vi "Auto_Path Tracking_KBS.vi"() -> ()   [LabVIEW 2020]
uses:
  <vilib>/Utility/file.llb/Read Delimited Spreadsheet (DBL).vi
  <vilib>/Instr/_visa.llb/VISA Configure Serial Port (Instr).vi
panel:
  out "Tracking_Error(m)":dbl
  out "TM_X(lat)":dbl format="%-#_10g M"
  out "TM_Y(long)":dbl format="%-#_10g M"
  out "F9P_Data_GPGGA_Raw":string
  out "GPS_KHP":dbl
  out "Heading_T":dbl
  out "Heading_M":dbl
  out "F9P GPS Data":T1
  in  "COM":refnum<visa-resource-name>="COM4"
  in  "?":enum32{"State", "ETC"}(tab)
  in  "stop":bool
  in  "file path (dialog if empty)":path caption="RDDF"
  out "XY Graph":T2(graph)
  in  "Refresh":bool
  in  "A/M":bool=TRUE
  in  "Serial Name":refnum<visa-resource-name>="COM8"
  out "ERP_Serial_DATA(RAW)":string
  in  "Vel":dbl=4.0 format="%#_13g"
  out "Index(near vehicle)":i32
  out "WP_no.":i32
  out "x_lat_path":dbl[](array[numeric])
  out "y_long_path":dbl[](array[numeric])
  out "vel. path":dbl[](array[numeric])
  out "Path_Vel_arr":dbl[](array[numeric])
  out "Path_long_arr":dbl[](array[numeric])
  out "Path_lat_arr":dbl[](array[numeric])
  out "ERP_Receive":T3
  out "Steer_CMD(Deg)":dbl
  out "CMD_2_ERP":T4
  out "Brake":u8
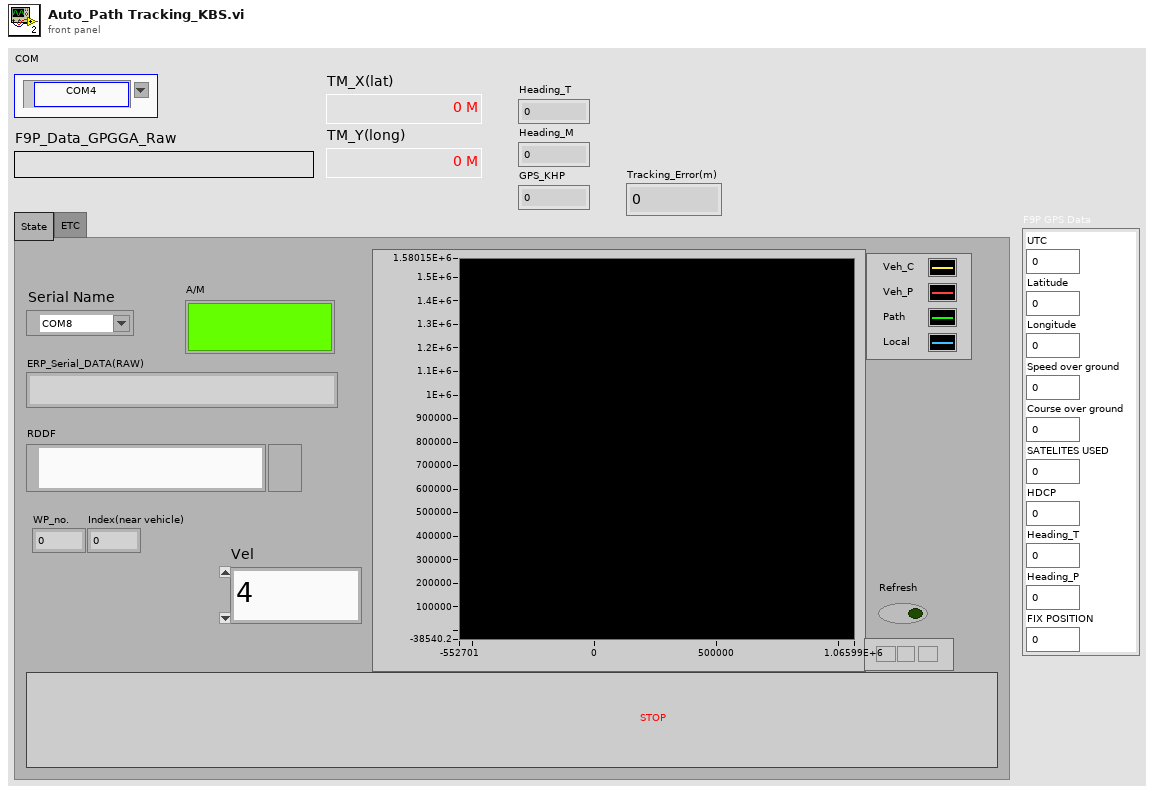
[diagram p1: front panel]
types:
  T1 = cluster{"UTC":dbl, "Latitude":dbl, "Longitude":dbl, "Speed over ground":dbl, "Course over ground":dbl, "SATELITES USED":i32, "HDCP":dbl, "Heading_T":dbl, "Heading_P":dbl, "FIX POSITION":i32}
  T2 = cluster{"y_long_path":dbl[], "x_lat_path":dbl[]}[]
  T3 = cluster{"AorM":u8, "E-Stop":u8, "F_B":u8, "Speed":u16, "Steer":i16, "Brake":u8, "Encoder":u8, "Encoder 2":u8, "Encoder 3":u8, "Encoder 4":u8, "ALIVE":u8, "ETX_0":u8, "ETX_0 2":u8}
  T4 = cluster{"F/B":u8, "Speed":u16, "Steer":i16, "A/M":u8, "Brake":u8}
  T5 = cluster{"Path_long_arr":dbl[], "Path_lat_arr":dbl[]}
  T6 = cluster{"Path_long_arr":dbl[], "Path_lat_arr":dbl[]}[]
  T7 = cluster{"S":u8, "T":u8, "X":u8, "AorM":u8, "E-Stop":u8, "F_B":u8, "Speed":u16, "Steer":i16, "Brake":u8, "ALIVE":u8, "ETX_0":u8, "ETX_0 2":u8}
  T8 = cluster{"UTC":dbl, "Latitude":dbl, "N/S":i8, "Longitude":dbl, "N/S":i8, "FIX POSITION":i32, "SATELITES USED":i32, "HDCP":dbl}
  T9 = cluster{"UTC":dbl, "N/S":i8, "Latitude":dbl, "N/S 2":i8, "Longitude":dbl, "N/S 3":i8, "Speed over ground":dbl, "Course over ground":dbl}
  T10 = cluster{"Heading_T":dbl, "T":i8, "Heading_M":dbl, "M":i8, "G_Speed_Knote":dbl, "N":i8, "G_Speed_KPH":dbl}
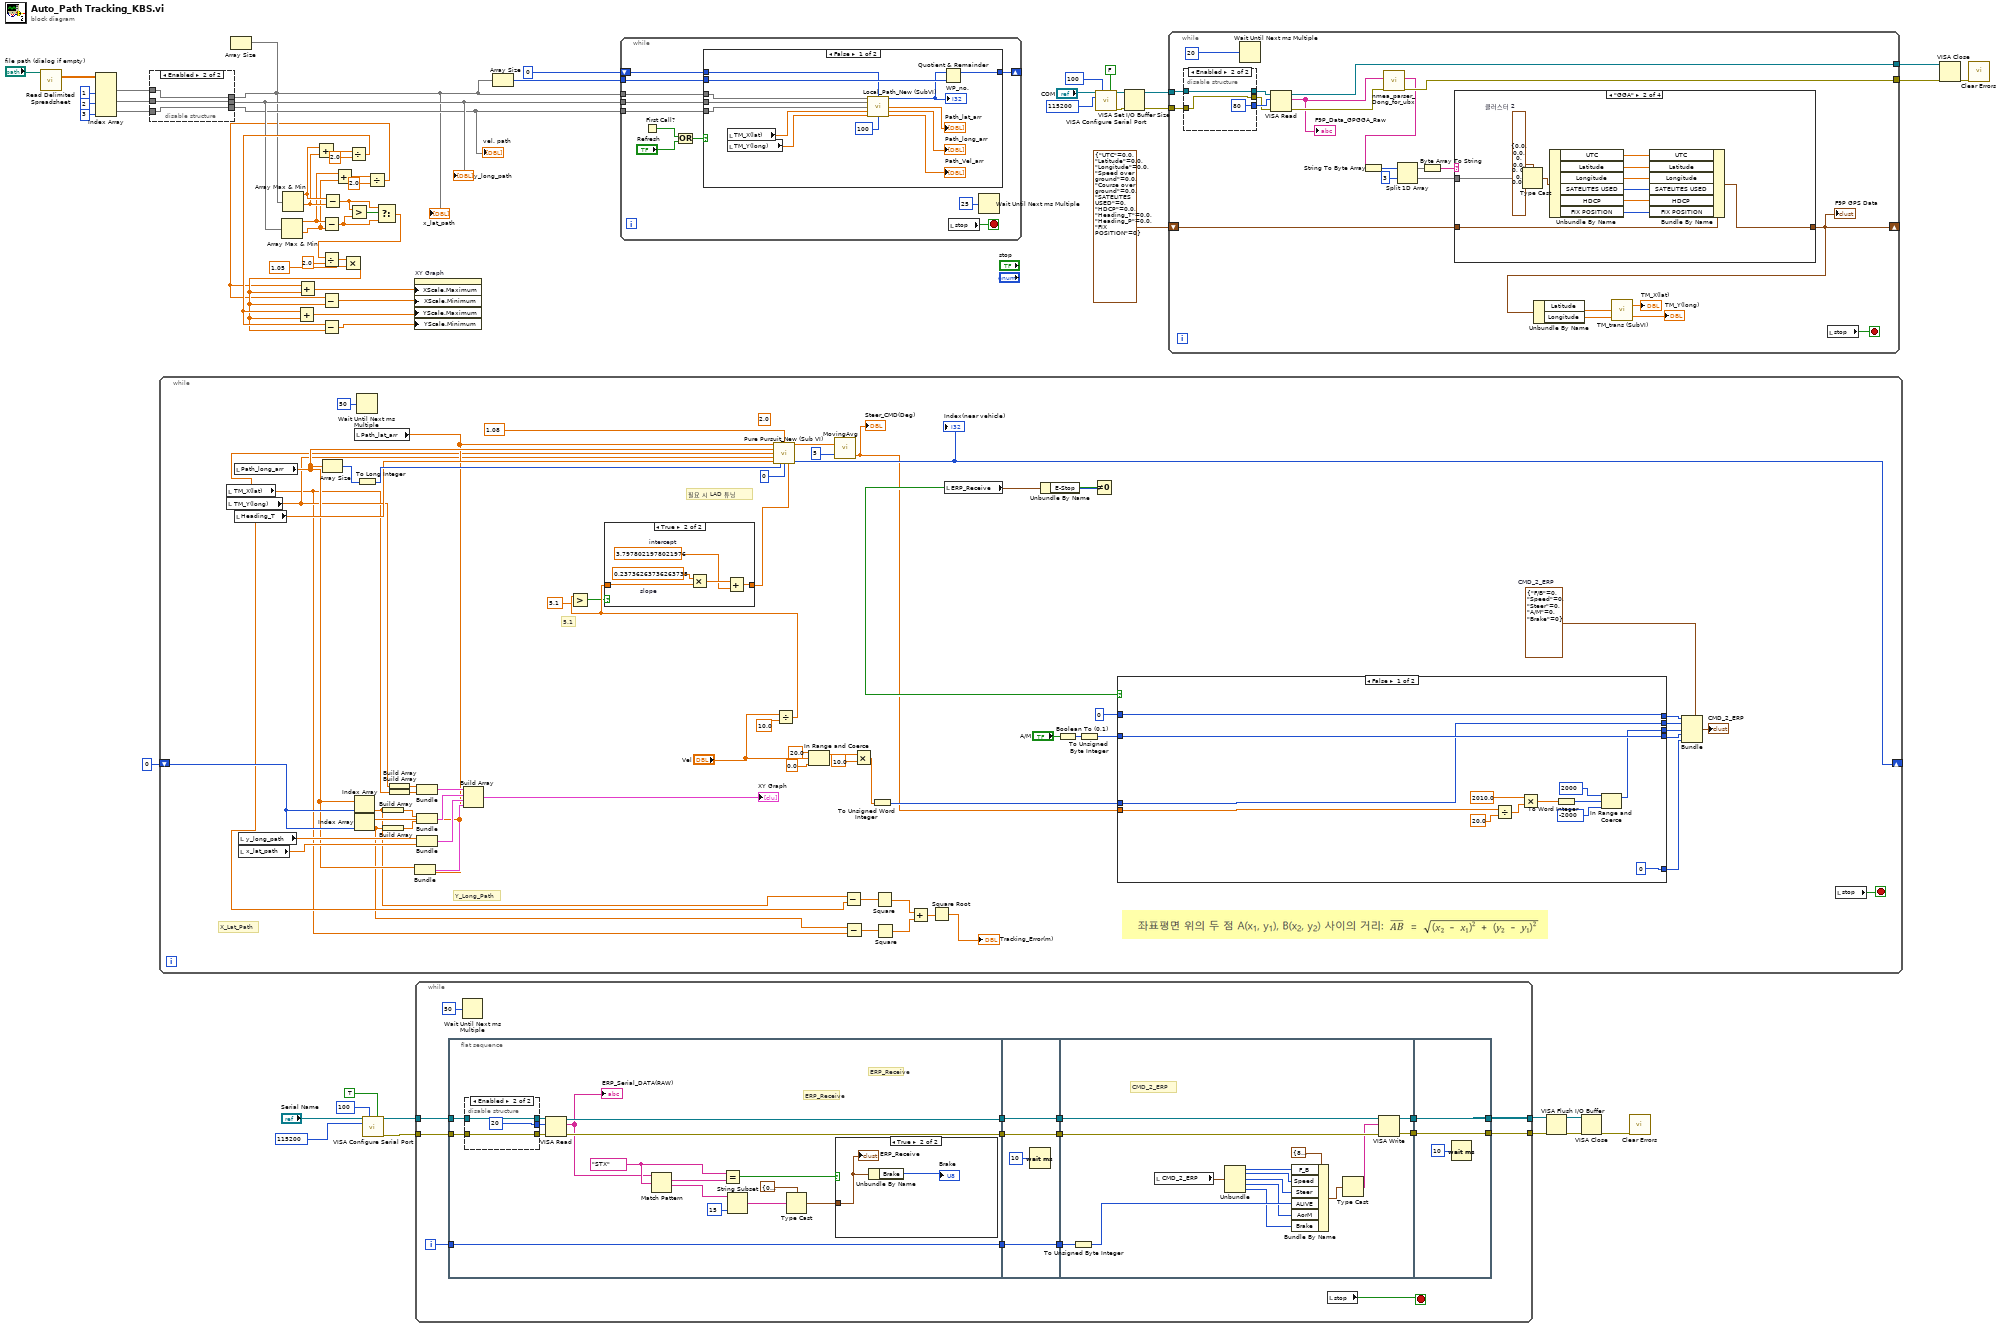
[diagram p0: block diagram]
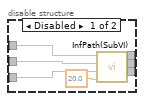
[diagram p2: hidden frame]
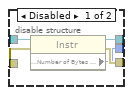
[diagram p3: hidden frame]
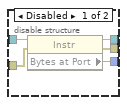
[diagram p5: hidden frame]
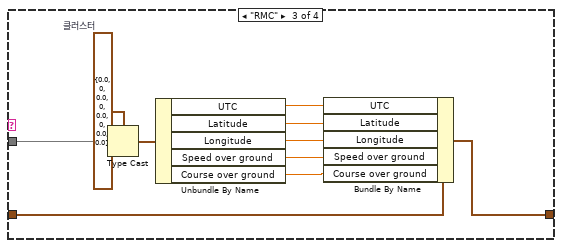
[diagram p7: hidden frame]
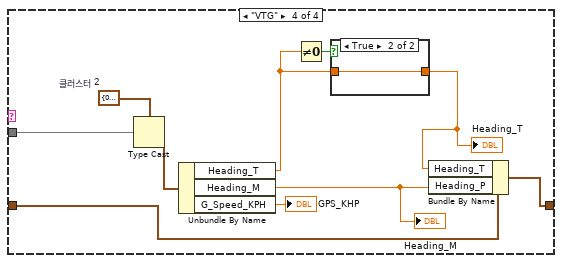
[diagram p8: hidden frame]
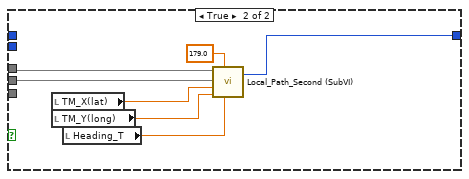
[diagram p10: hidden frame]
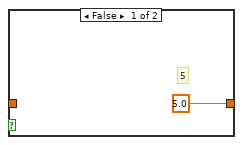
[diagram p11: hidden frame]
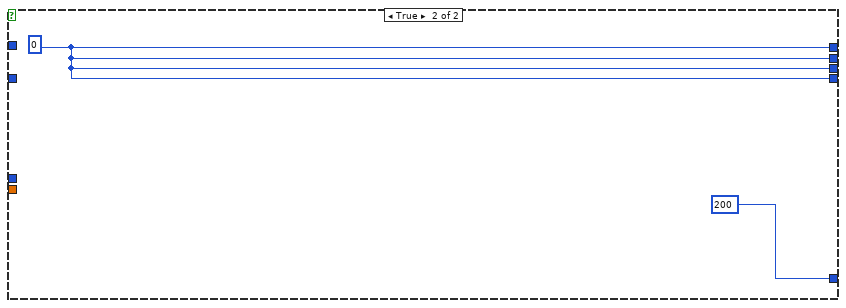
[diagram p12: hidden frame]
diagram:
  n1 = call-poly <vilib>:"Read Delimited Spreadsheet.vi"("file path (dialog if empty)"="file path (dialog if empty)") -> ("all rows"=w27:dbl[][])  [unwired: 9 in, 5 out]
  n2 = Index Array(array=w27, index (col) #1=1 ("비활성화된 인덱스 (열)"), index (col) #2=2 ("인덱스 (열)"), index (col) #3=3 ("인덱스 (열)")) -> (element #1=w56:dbl[], element #2=w55:dbl[], element #3=w54:dbl[])  [unwired: 3 in]
  n3 = disable-structure shown="Enabled" {
    disable-tunnel: w56 -> [w66 w69]
    disable-tunnel: w55 -> [w65 w68]
    disable-tunnel: w54 -> [w64 w67]
    disable-tunnel: [w63 w68] -> w31
    disable-tunnel: [w62 w67] -> w29
    disable-tunnel: [w61 w69] -> w28
    frame Disabled {
      n4 = call "InfPath(SubVI).vi"("Mod dist."=20.0, "vel."=w64, "y_long"=w65, "x_lat"=w66) -> ("vel. path"=w62:dbl[], "y_long_path"=w63:dbl[], "x_lat_path"=w61:dbl[])  [unwired: 1 out]
    }
    frame Enabled {
    }
  }
  "x_lat_path" <- w28
  "y_long_path" <- w31
  "vel. path" <- w29
  n5 = while {
    shift-right: [w117] -> _
    shift-left: 0 -> [w114]
    stop <- w123 stop-if-true
    w89 = T4 {"F/B"=0, "Speed"=0, "Steer"=0, "A/M"=0, "Brake"=0}  # CMD_2_ERP
    (unwired) 2.0 ("L")
    # "5.1"
    # "X_Lat_Path"
    # "Y_Long_Path"
    # "필요 시 LAD 튜닝"
    n6 = local read "TM_X(lat)"() -> (w83:dbl)
    n7 = local read "TM_Y(long)"() -> (w84:dbl)
    n8 = local read "Path_long_arr"() -> (w86:dbl[])
    n9 = local read "Heading_T"() -> (w110:dbl)
    n10 = local read "y_long_path"() -> (w94:dbl[])
    n11 = local read "x_lat_path"() -> (w93:dbl[])
    n12 = Array Size(array=w86) -> (size(s)=w118:i32)
    n13 = local read "Path_lat_arr"() -> (w85:dbl[])
    n14 = Index Array(array=w86, index=w114) -> (element=w74:dbl)
    n15 = Index Array(array=w85, index=w114) -> (element=w73:dbl)
    n16 = Wait Until Next ms Multiple(millisecond multiple=u32 50 ("ms 배수")) -> ()  [unwired: 1 out]
    n17 = To Long Integer(number=w118) -> (32bit integer=w116:i32)
    n18 = Build Array(w74) -> (w125:dbl[])
    n19 = Build Array(w73) -> (w124:dbl[])
    n20 = Build Array(w84) -> (w127:dbl[])
    n21 = Build Array(w83) -> (w126:dbl[])
    n22 = Bundle("Path_long_arr"=w86, "Path_lat_arr"=w85) -> (w106:T5)  [unwired: 1 in]
    n23 = Bundle(w127, w126) -> (w112:cluster{dbl[], dbl[]})  [unwired: 1 in]
    n24 = Bundle(w125, w124) -> (w111:cluster{dbl[], dbl[]})  [unwired: 1 in]
    n25 = Bundle("y_long_path"=w94, "x_lat_path"=w93) -> (w113:cluster{"y_long_path":dbl[], "x_lat_path":dbl[]})  [unwired: 1 in]
    n26 = Build Array(w112, w111, w113, w106) -> (→"XY Graph":T6)
    n27 = Divide(x="Vel", y=10.0) -> (x/y=w107:dbl)
    n28 = Greater?(x=w107, y=5.1) -> (0:w72:bool)
    n29 = case shown="True" w72 {
      tunnel: w107 -> [_ w133]
      tunnel: [5.0 w132] -> w109
      frame False {
        # "5"
      }
      frame True {
        w134 = 3.7978021978021976  # intercept
        w136 = 0.23736263736263735  # slope
        n30 = Multiply(x=w136, y=w133) -> (x*y=w135:dbl)
        n31 = Add(x=w135, y=w134) -> (x+y=w132:dbl)
      }
    }
    n32 = call "Pure Pursuit_New (Sub VI).vi"("x_lat_path"=w85, "L"=1.08, "y_long_path"=w86, "X_Current"=w83, "Y_Current"=w84, "Heading_Current"=w110, "#pnt"=w116, "WP no_pre"=0, "LAD"=w109) -> ("Steer_CMD(Deg)"=w82:dbl, "Index(near vehicle)"=w117:i32)  [unwired: 5 in]
    "Index(near vehicle)" <- w117
    n33 = In Range and Coerce(upper limit=20.0 ("상위 리미트"), x="Vel", lower limit=0.0 ("하위 리미트")) -> (coerced(x)=w98:dbl)  [unwired: 1 out]
    n34 = call "MovingAvg.vi"("입력"=w82, "이동평균을 구할 자료의 개수"=u16 5) -> ("이동평균"=w70:dbl)  [unwired: 2 out]
    "Steer_CMD(Deg)" <- w70
    n35 = Subtract(x=w74, y=w84) -> (x-y=w79:dbl)
    n36 = Subtract(x=w73, y=w83) -> (x-y=w78:dbl)
    n37 = Multiply(x=w98, y=10.0) -> (x*y=w96:dbl)
    n38 = To Unsigned Word Integer(number=w96) -> (unsigned 16bit integer=w102:u16)
    n39 = Square(x=w79) -> (x^2=w77:dbl)
    n40 = Square(x=w78) -> (x^2=w76:dbl)
    n41 = Add(x=w77, y=w76) -> (x+y=w75:dbl)
    n42 = Square Root(x=w75) -> (sqrt(x)=→"Tracking_Error(m)":dbl)
    n43 = local read "ERP_Receive"() -> (w120:T3)
    n44 = Unbundle By Name(w120) -> ("E-Stop"=w121:u8)
    n45 = Boolean To (0,1)(Boolean="A/M") -> (0, 1=w105:i16)
    n46 = To Unsigned Byte Integer(number=w105) -> (unsigned 8bit integer=w87:u8)
    n47 = Not Equal To 0?(x=w121) -> (x != 0?=w101:bool)
    n48 = case shown="False" w101 {
      tunnel: u8 0 -> [w149 _]
      tunnel: [w149 w151] -> w130
      tunnel: [w146 w151] -> w129
      tunnel: [w138 w151] -> w128
      tunnel: [w148 w151] -> w104
      tunnel: w87 -> [w148 _]
      tunnel: w70 -> [w147 _]
      tunnel: w102 -> [w146 _]
      tunnel: [u8 0 u8 200] -> w90
      frame False {
        n49 = Divide(x=w147, y=20.0) -> (x/y=w144:dbl)
        n50 = Multiply(x=2010.0, y=w144) -> (x*y=w143:dbl)
        n51 = To Word Integer(number=w143) -> (16bit integer=w145:i16)
        n52 = In Range and Coerce(upper limit=i16 2000 ("상위 리미트"), x=w145, lower limit=i16 -2000 ("하위 리미트")) -> (coerced(x)=w138:i16)  [unwired: 1 out]
      }
      frame True {
        w151 = u8 0
      }
    }
    n53 = Bundle(cluster=w89, "F/B"=w130, "Speed"=w129, "Steer"=w128, "A/M"=w104, "Brake"=w90) -> (→"CMD_2_ERP":T4)
    n54 = local read "stop"() -> (w123:bool)
  }
  n55 = Array Size(array=w28) -> ()  [unwired: 1 out]
  n56 = Array Max & Min(array=w31) -> (max value=w42:dbl, min value=w41:dbl)  [unwired: 2 out]
  n57 = Array Max & Min(array=w28) -> (max value=w48:dbl, min value=w47:dbl)  [unwired: 2 out]
  n58 = Add(x=w48, y=w47) -> (x+y=w45:dbl)
  n59 = Subtract(x=w42, y=w41) -> (x-y=w51:dbl)
  n60 = Subtract(x=w48, y=w47) -> (x-y=w52:dbl)
  n61 = Add(x=w42, y=w41) -> (x+y=w44:dbl)
  n62 = Divide(x=w45, y=2.0) -> (x/y=w38:dbl)
  n63 = Greater?(x=w52, y=w51) -> (0:w53:bool)
  n64 = call-poly "VISA Configure Serial Port"("VISA resource name"="Serial Name", "timeout (10sec)"=u32 100, "Enable Termination\nChar (T)"=TRUE ("Enable Termination\nChar (T)"), "baud rate (9600)"=u32 115200) -> ("VISA resource name out"=w3:refnum<visa-resource-name>, "error out"=w2:errorcluster)  [unwired: 10 in]
  n65 = Divide(x=w44, y=2.0) -> (x/y=w25:dbl)
  n66 = Select(t=w52, s=w53, f=w51) -> (s? t:f=w49:dbl)
  n67 = Divide(x=w49, y=2.0) -> (x/y=w40:dbl)
  n68 = Multiply(x=w40, y=1.05) -> (x*y=w37:dbl)
  n69 = Add(x=w38, y=w37) -> (x+y=w35:dbl)
  n70 = Add(x=w25, y=w37) -> (x+y=w33:dbl)
  n71 = Subtract(x=w25, y=w37) -> (x-y=w34:dbl)
  n72 = Subtract(x=w38, y=w37) -> (x-y=w36:dbl)
  n73 = property on="XY Graph" class="XYGraph (strict)"("XScale.Maximum"=w33, "XScale.Minimum"=w34, "YScale.Maximum"=w35, "YScale.Minimum"=w36) -> ()  [unwired: 2 in, 2 out]
  n74 = while {
    tunnel: w3 -> [w165]
    tunnel: w2 -> [w164]
    tunnel: [w162] -> w5
    tunnel: [w161] -> w4
    i -> [w163]
    stop <- w154 stop-if-true
    n75 = flat-sequence {
      tunnel: w165 -> [w183]
      tunnel: w164 -> [w182]
      tunnel: [w181] -> w160
      tunnel: [w180] -> w158
      tunnel: w163 -> [w179]
      tunnel: [w179] -> w156
      tunnel: w160 -> [w197]
      tunnel: [w197] -> w159
      tunnel: w158 -> [w196]
      tunnel: [w196] -> w157
      tunnel: w156 -> [w195]
      tunnel: [w195] -> w155
      tunnel: w159 -> [w210]
      tunnel: w157 -> [w209]
      tunnel: w155 -> [w207]
      tunnel: [w206] -> w153
      tunnel: [w205] -> w152
      tunnel: [w214] -> w161
      tunnel: [w215] -> w162
      tunnel: w153 -> [w215]
      tunnel: w152 -> [w214]
      frame #0 {
        w173 = "STX" ("검색 문자열/문자 (-)")
        # "ERP_Receive"
        # "ERP_Receive"
        n76 = disable-structure shown="Enabled" {
          disable-tunnel: w183 -> [w188 w190]
          disable-tunnel: w182 -> [w187 w191]
          disable-tunnel: [w186 w191] -> w178
          disable-tunnel: [w185 u32 20 ("timeout (10sec)")] -> w177
          disable-tunnel: [w184 w190] -> w176
          frame Disabled {
            n77 = property class="Instr"(reference=w188, error in=w187) -> (reference out=w184:refnum<visa-resource-name>, error out=w186:errorcluster, "Serial Settings:Number of Bytes at Serial Port"=w185:u32)
          }
          frame Enabled {
          }
        }
        n78 = VISA Read(VISA resource name=w176, byte count=w177, error in (no error)=w178) -> (VISA resource name out=w181:refnum<visa-resource-name>, read buffer=w171:string, error out=w180:errorcluster)  [unwired: 1 out]
        "ERP_Serial_DATA(RAW)" <- w171
        n79 = Match Pattern(string=w171, regular expression=w173) -> (match substring=w172:string, after substring=w175:string)  [unwired: 1 in, 2 out]
        n80 = Equal?(x=w173, y=w172) -> (x = y?=w170:bool)
        n81 = String Subset(string=w175, length (rest)=15 ("길이(나머지)")) -> (substring=w169:string)  [unwired: 1 in]
        n82 = Type Cast(type=T3 {"AorM"=0, "E-Stop"=0, "F_B"=0, "Speed"=0, "Steer"=0, "Brake"=0, "Encoder"=0, "Encoder 2"=0, "Encoder 3"=0, "Encoder 4"=0, "ALIVE"=0, "ETX_0"=13, "ETX_0 2"=10}, x=w169) -> (*(type *) &x=w168:T3)
        n83 = case shown="True" w170 {
          tunnel: w168 -> [_ w193]
          frame False {
          }
          frame True {
            n84 = Unbundle By Name(w193) -> ("Brake"=→"Brake":u8)
            "ERP_Receive" <- w193
          }
        }
      }
      frame #1 {
        n85 = Wait (ms)(milliseconds to wait=u32 10 ("대기 시간(ms)")) -> ()  [unwired: 1 out]
      }
      frame #2 {
        # "CMD_2_ERP"
        n86 = To Unsigned Byte Integer(number=w207) -> (unsigned 8bit integer=w212:u8)
        n87 = local read "CMD_2_ERP"() -> (w199:T4)
        n88 = Unbundle(w199) -> ("F/B"=w204:u8, "Speed"=w203:u16, "Steer"=w202:i16, "A/M"=w200:u8, "Brake"=w198:u8)
        n89 = Bundle By Name(cluster=T7 {"S"=83, "T"=84, "X"=88, "AorM"=0, "E-Stop"=0, "F_B"=0, "Speed"=0, "Steer"=0, "Brake"=0, "ALIVE"=0, "ETX_0"=13, "ETX_0 2"=10}, "F_B"=w204, "Speed"=w203, "Steer"=w202, "ALIVE"=w212, "AorM"=w200, "Brake"=w198) -> (w211:T7)
        n90 = Type Cast(x=w211) -> (*(type *) &x=w208:string)  [unwired: 1 in]
        n91 = VISA Write(VISA resource name=w210, write buffer=w208, error in (no error)=w209) -> (VISA resource name out=w206:refnum<visa-resource-name>, error out=w205:errorcluster)  [unwired: 1 out]
      }
      frame #3 {
        n92 = Wait (ms)(milliseconds to wait=u32 10 ("대기 시간(ms)")) -> ()  [unwired: 1 out]
      }
    }
    n93 = Wait Until Next ms Multiple(millisecond multiple=u32 50 ("ms 배수")) -> ()  [unwired: 1 out]
    n94 = local read "stop"() -> (w154:bool)
  }
  n95 = Array Size(array=w28) -> (size(s)=w30:i32)
  n96 = while {
    tunnel: w28 -> [w225]
    tunnel: w31 -> [w224]
    tunnel: w29 -> [w222]
    tunnel: w30 -> [w221]
    shift-right: [w220] -> _
    shift-left: 0 ("Index0") -> [w223]
    stop <- w226 stop-if-true
    n97 = First Call?() -> (First Call?: T/F=w218:bool)
    n98 = Or(x=w218, y="Refresh") -> (x .or. y?=w219:bool)
    n99 = case shown="False" w219 {
      tunnel: w225 -> [w227 w246]
      tunnel: w224 -> [w229 w245]
      tunnel: w223 -> [w234 _]
      tunnel: w222 -> [w228 _]
      tunnel: w221 -> [w238 _]
      tunnel: [w239 w240] -> w220
      frame False {
        n100 = local read "TM_X(lat)"() -> (w237:dbl)
        n101 = local read "TM_Y(long)"() -> (w236:dbl)
        n102 = call "Local_Path_New (SubVI).vi"("x_lat_arr"=w227, "WP no_pre"=w234, "y_long_arr"=w229, "vel_arr"=w228, "x_lat_c"=w237, "y_long_c"=w236, "# of pnt"=100) -> ("INDEX(Near Point)"=w230:i32, "Lat(Local)"=→"Path_lat_arr":dbl[], "Long(Local)"=→"Path_long_arr":dbl[], "Vel(Local)"=→"Path_Vel_arr":dbl[])  [unwired: 5 in]
        "WP_no." <- w230
        n103 = Quotient & Remainder(x=w230, y=w238) -> (x-y*floor(x/y)=w239:i32)  [unwired: 1 out]
      }
      frame True {
        n104 = local read "TM_X(lat)"() -> (w244:dbl)
        n105 = local read "TM_Y(long)"() -> (w243:dbl)
        n106 = local read "Heading_T"() -> (w242:dbl)
        n107 = call "Local_Path_Second (SubVI).vi"("heading_deg"=w242, "heading_limit"=179.0, "y_long"=w243, "x_lat"=w244, "Y_long_path"=w245, "X_lat_path"=w246) -> ("Index(near vehicle)"=w240:i32)  [unwired: 1 out]
      }
    }
    n108 = local read "stop"() -> (w226:bool)
    n109 = Wait Until Next ms Multiple(millisecond multiple=u32 25) -> ()  [unwired: 1 out]
  }
  n110 = call-poly "VISA Configure Serial Port"("VISA resource name"="COM", "timeout (10sec)"=u32 100, "Enable Termination\nChar (T)"=FALSE ("Enable Termination\nChar (T)"), "baud rate (9600)"=u32 115200 ("baud rate")) -> ("VISA resource name out"=w20:refnum<visa-resource-name>, "error out"=w19:errorcluster)  [unwired: 10 in]
  n111 = VISA Set I/O Buffer Size(VISA resource name=w20, error in (no error)=w19) -> (VISA resource name out=w15:refnum<visa-resource-name>, error out=w14:errorcluster)  [unwired: 2 in]
  n112 = while {
    shift-right: [w261] -> _
    shift-left: T1 {"UTC"=0.0, "Latitude"=0.0, "Longitude"=0.0, "Speed over ground"=0.0, "Course over ground"=0.0, "SATELITES USED"=0, "HDCP"=0.0, "Heading_T"=0.0, "Heading_P"=0.0, "FIX POSITION"=0} ("Garmin GPS Data") -> [w269]
    tunnel: w15 -> [w253]
    tunnel: w14 -> [w251]
    tunnel: [w262] -> w18
    tunnel: [w268] -> w17
    stop <- w248 stop-if-true
    n113 = disable-structure shown="Enabled" {
      disable-tunnel: [w274 u32 80 ("Bytes at Port")] -> w254
      disable-tunnel: w253 -> [w273 w276]
      disable-tunnel: [w272 w276] -> w252
      disable-tunnel: w251 -> [w271 w275]
      disable-tunnel: [w270 w275] -> w250
      frame Disabled {
        n114 = property class="Instr"(reference=w273, error in=w271) -> (reference out=w272:refnum<visa-resource-name>, error out=w270:errorcluster, "Bytes at Port"=w274:u32)
      }
      frame Enabled {
      }
    }
    n115 = Wait Until Next ms Multiple(millisecond multiple=u32 20 ("타임아웃(ms) (-1)")) -> ()  [unwired: 1 out]
    n116 = VISA Read(VISA resource name=w252, byte count=w254, error in (no error)=w250) -> (VISA resource name out=w262:refnum<visa-resource-name>, read buffer=w263:string, error out=w267:errorcluster)  [unwired: 1 out]
    "F9P_Data_GPGGA_Raw" <- w263
    n117 = call "nmea_parser_Dong_for_ubx.vi"("error in"=w267, "INPUT"=w263) -> ("error out"=w268:errorcluster, "output"=w255:string)  [unwired: 8 in]
    n118 = String To Byte Array(string=w255) -> (unsigned byte array=w259:u8[])
    n119 = Split 1D Array(array=w259, index=3) -> (first subarray=w258:u8[], second subarray=w257:u8[])
    n120 = Byte Array To String(unsigned byte array=w258) -> (string=w256:string)
    n121 = case shown="\"GGA\"" w256 {
      tunnel: w257 -> [_ w289 w297 w309]
      tunnel: w269 -> [w278 w285 w296 w305]
      tunnel: [w278 w284 w295 w306] -> w261
      frame Default {
      }
      frame "GGA" {
        w287 = T8 {"UTC"=0.0, "Latitude"=0.0, "N/S"=0, "Longitude"=0.0, "N/S"=0, "FIX POSITION"=0, "SATELITES USED"=0, "HDCP"=0.0}  # 클러스터 2
        n122 = Type Cast(type=w287, x=w289) -> (*(type *) &x=w288:T8)
        n123 = Unbundle By Name(w288) -> ("UTC"=w286:dbl, "Latitude"=w283:dbl, "Longitude"=w282:dbl, "SATELITES USED"=w281:i32, "HDCP"=w280:dbl, "FIX POSITION"=w279:i32)
        n124 = Bundle By Name(cluster=w285, "UTC"=w286, "Latitude"=w283, "Longitude"=w282, "SATELITES USED"=w281, "HDCP"=w280, "FIX POSITION"=w279) -> (w284:T1)
      }
      frame "RMC" {
        w299 = T9 {"UTC"=0.0, "N/S"=0, "Latitude"=0.0, "N/S 2"=0, "Longitude"=0.0, "N/S 3"=0, "Speed over ground"=0.0, "Course over ground"=0.0}  # 클러스터
        n125 = Type Cast(type=w299, x=w297) -> (*(type *) &x=w298:T9)
        n126 = Unbundle By Name(w298) -> ("UTC"=w294:dbl, "Latitude"=w293:dbl, "Longitude"=w292:dbl, "Speed over ground"=w291:dbl, "Course over ground"=w290:dbl)
        n127 = Bundle By Name(cluster=w296, "UTC"=w294, "Latitude"=w293, "Longitude"=w292, "Speed over ground"=w291, "Course over ground"=w290) -> (w295:T1)
      }
      frame "VTG" {
        w308 = T10 {"Heading_T"=0.0, "T"=0, "Heading_M"=0.0, "M"=0, "G_Speed_Knote"=0.0, "N"=0, "G_Speed_KPH"=0.0}  # 클러스터 2
        n128 = Type Cast(type=w308, x=w309) -> (*(type *) &x=w307:T10)
        n129 = Unbundle By Name(w307) -> ("Heading_T"=w304:dbl, "Heading_M"=w301:dbl, "G_Speed_KPH"=→"GPS_KHP":dbl)
        "Heading_M" <- w301
        n130 = Not Equal To 0?(x=w304) -> (x != 0?=w303:bool)
        n131 = case shown="True" w303 {
          tunnel: w304 -> [_ w310]
          tunnel: [_ w310] -> w300
          frame False {
          }
          frame True {
          }
        }
        "Heading_T" <- w300
        n132 = Bundle By Name(cluster=w305, "Heading_T"=w300, "Heading_P"=w301) -> (w306:T1)
      }
    }
    "F9P GPS Data" <- w261
    n133 = Unbundle By Name(w261) -> ("Latitude"=w266:dbl, "Longitude"=w247:dbl)
    n134 = call "TM_trans (SubVI).vi"("long"=w247, "lat"=w266) -> ("Y(long)"=→"TM_Y(long)":dbl, "X(lat)"=→"TM_X(lat)":dbl)  [unwired: 1 in]
    n135 = local read "stop"() -> (w248:bool)
  }
  n136 = VISA Flush I/O Buffer(VISA resource name=w5, error in (no error)=w4) -> (VISA resource name out=w6:refnum<visa-resource-name>, error out=w7:errorcluster)  [unwired: 1 in]
  n137 = VISA Close(VISA resource name=w6, error in (no error)=w7) -> (error out=w1:errorcluster)
  n138 = call <vilib>:"Clear Errors.vi"("error in (no error)"=w1) -> ()  [unwired: 5 in, 2 out]
  n139 = VISA Close(VISA resource name=w18, error in (no error)=w17) -> (error out=w13:errorcluster)
  n140 = call <vilib>:"Clear Errors.vi"("error in (no error)"=w13) -> ()  [unwired: 5 in, 2 out]
